vi "config.vi"() -> ()   [LabVIEW 2013]
uses:
  <vilib>/Utility/config.llb/NI_LVConfig.lvlib
panel:
  in  "选项卡控件":enum32{"操作步骤", "产品管理"}(tab)
  in  "第二段":T1
  in  "参数设定":string[][](table)
  in  "删除":bool
  in  "确定":bool
  in  "添加":bool
  in  "退出":bool
  in  "更新":bool
  in  "产品型号":string(combo)
  in  "操作步骤":T2
  in  "请输入添加的产品名称":string
  in  "请选择要删除的产品":string(combo)
  # "出厂检验台"
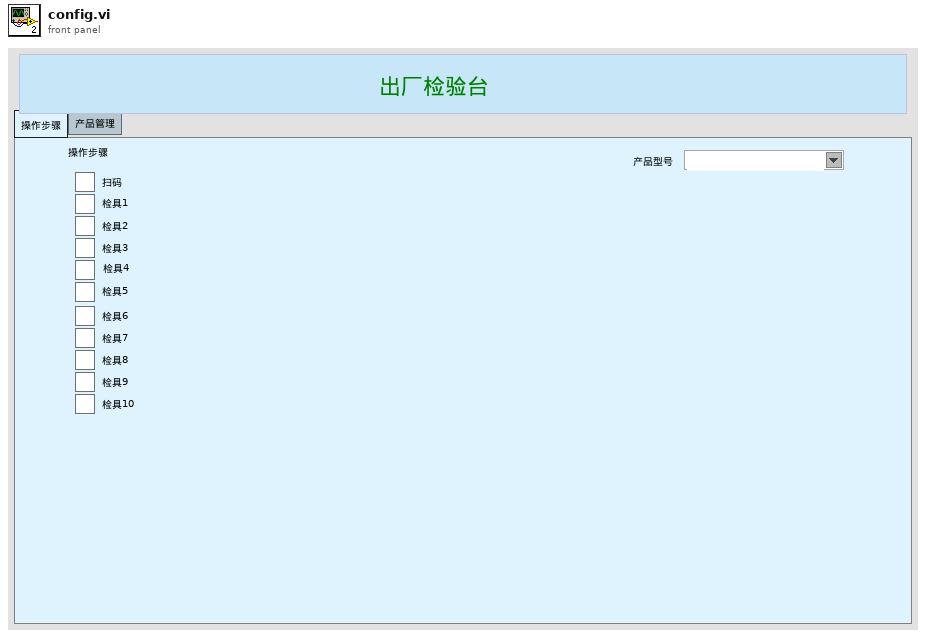
[diagram p1: front panel]
types:
  T1 = cluster{"检具6":bool, "检具7":bool, "检具8":bool, "检具9":bool, "检具10":bool}
  T2 = cluster{"扫码":bool, "检具1":bool, "检具2":bool, "检具3":bool, bool, "检具5":bool}
  T3 = typedef "NI_LVConfig.lvlib/Config Data RefNum.ctl" = refnum<k1>
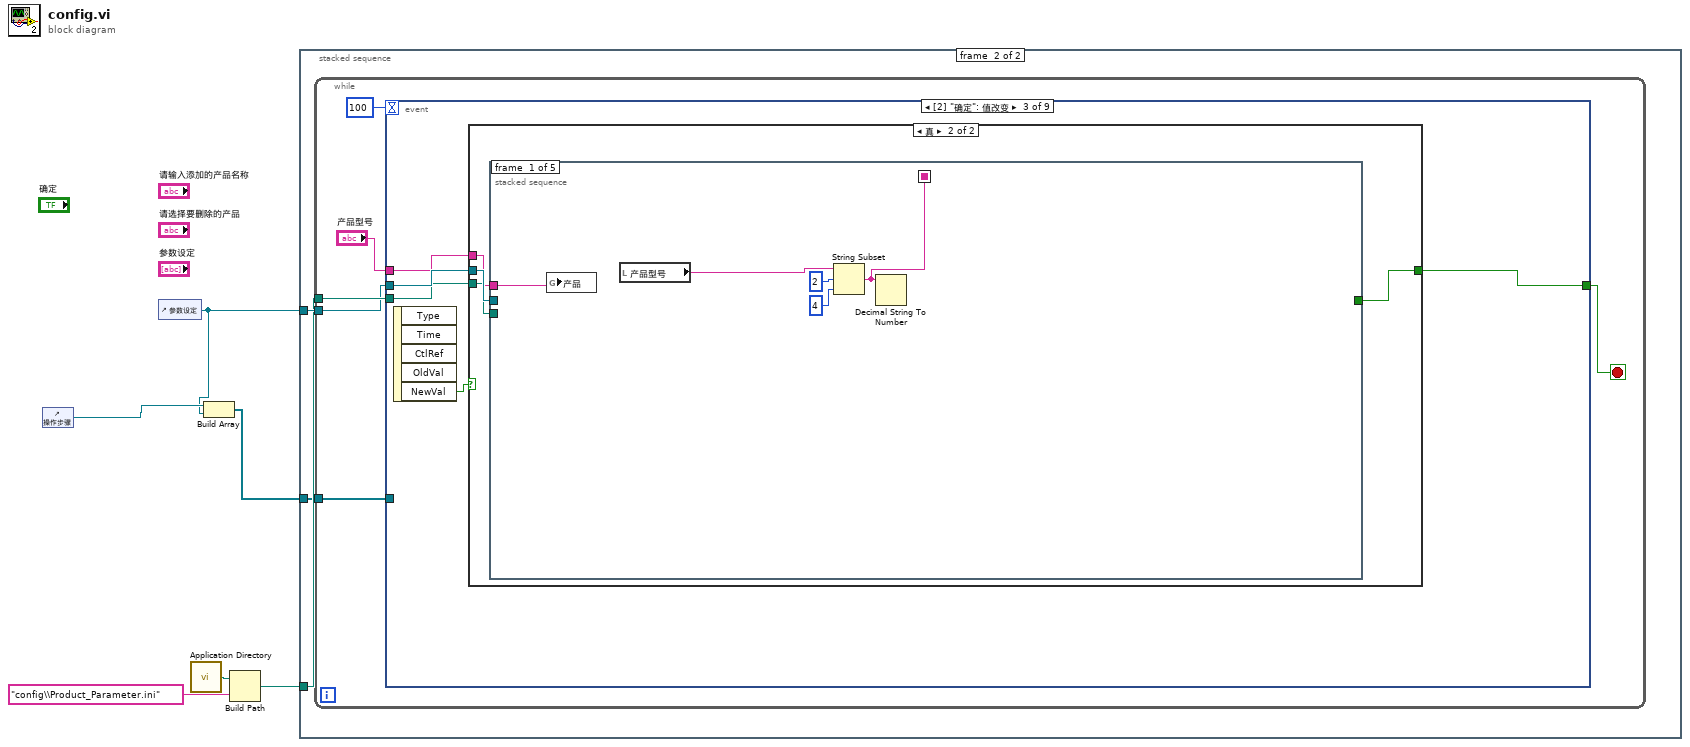
[diagram p0: block diagram]
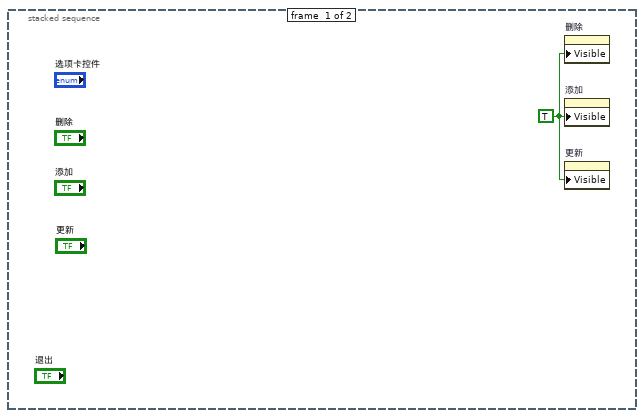
[diagram p2: hidden frame]
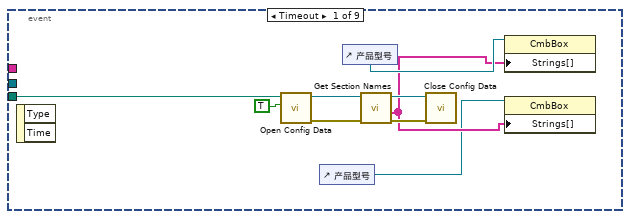
[diagram p3: hidden frame]
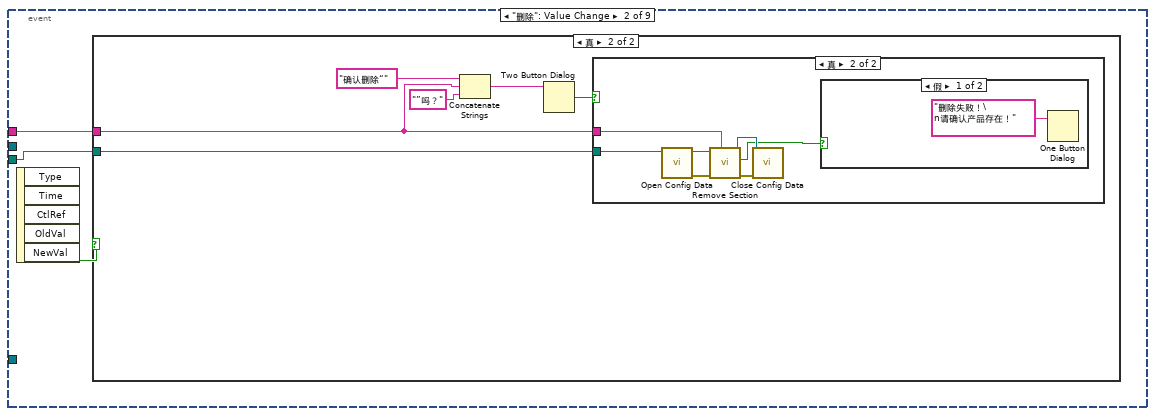
[diagram p4: hidden frame]
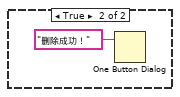
[diagram p7: hidden frame]
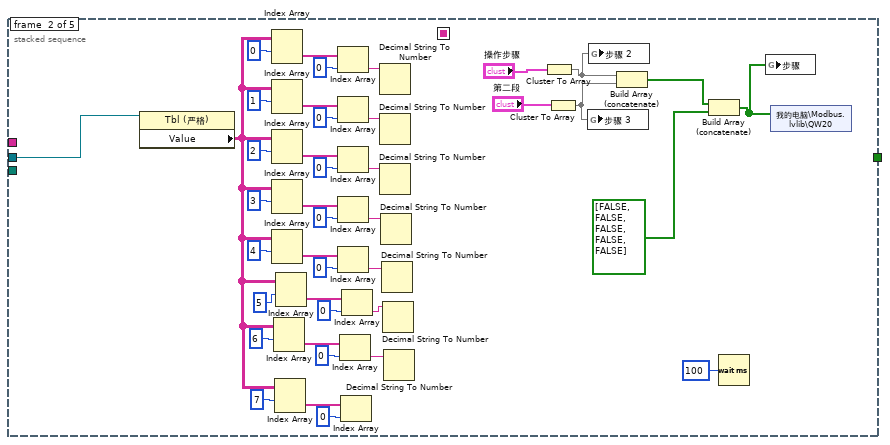
[diagram p9: hidden frame]
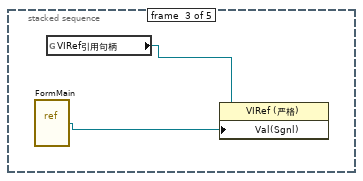
[diagram p10: hidden frame]
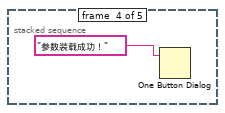
[diagram p11: hidden frame]
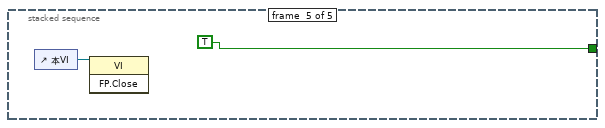
[diagram p12: hidden frame]
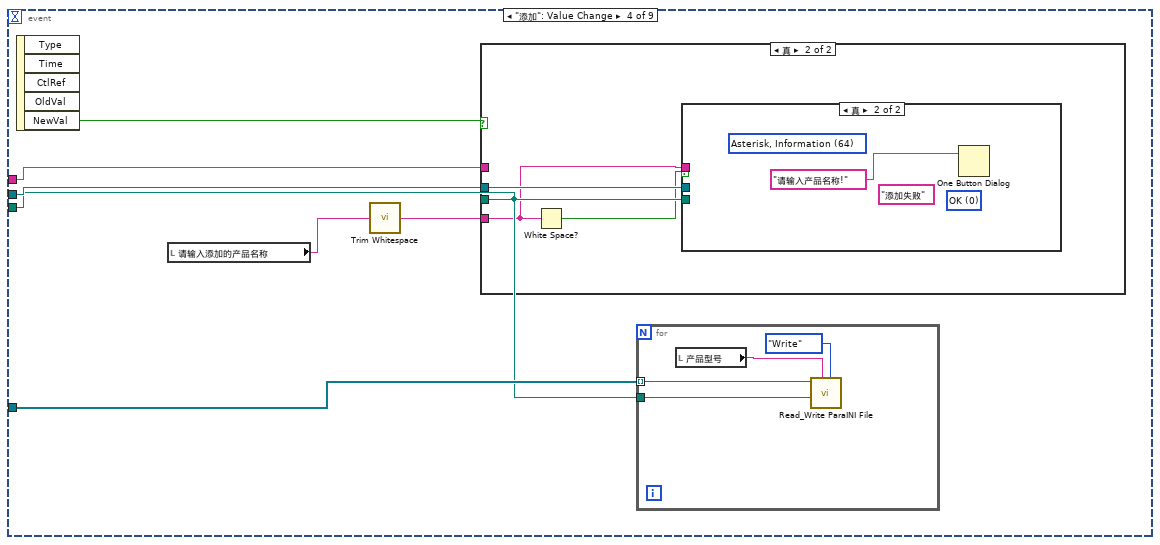
[diagram p13: hidden frame]
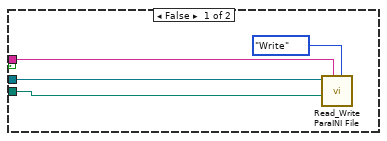
[diagram p15: hidden frame]
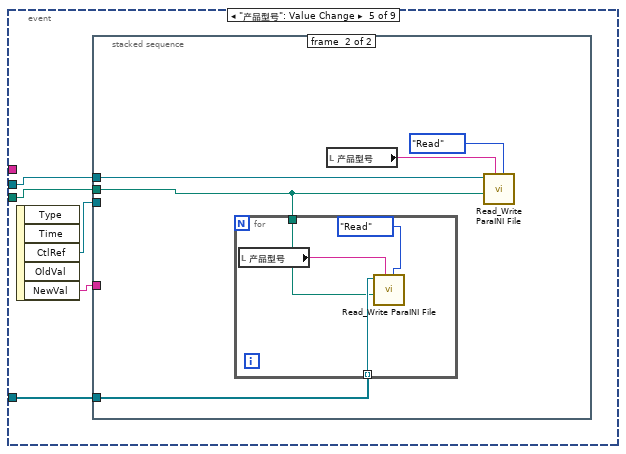
[diagram p16: hidden frame]
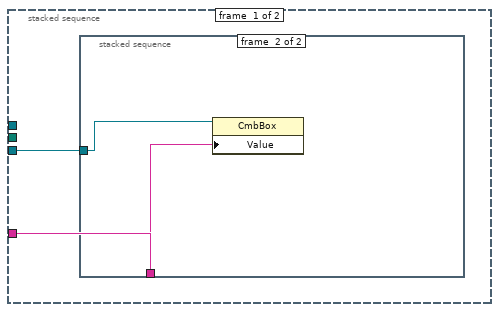
[diagram p17: hidden frame]
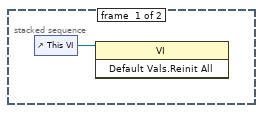
[diagram p18: hidden frame]
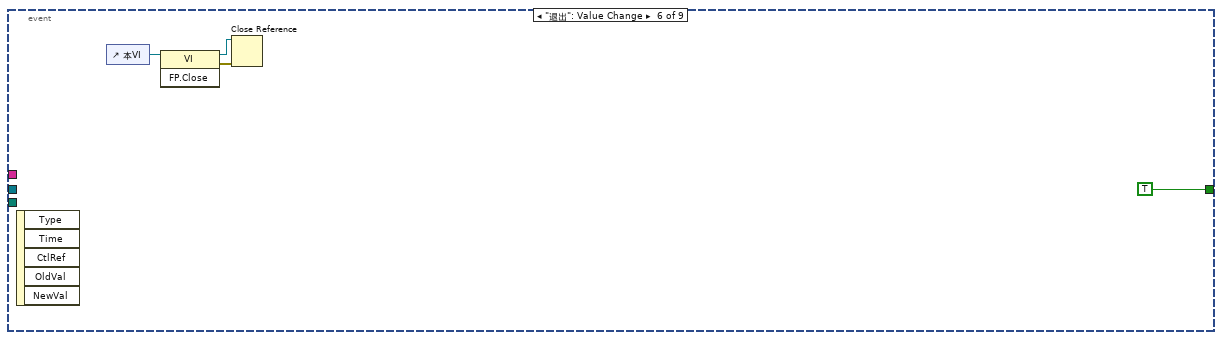
[diagram p19: hidden frame]
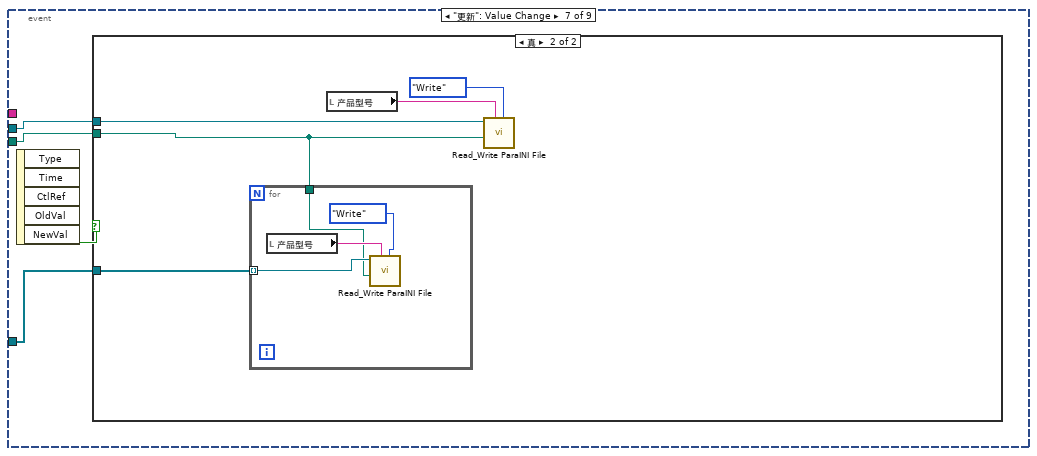
[diagram p20: hidden frame]
diagram:
  n1 = control-ref of="操作步骤"() -> (w3:refnum<vi>)
  n2 = control-ref of="参数设定"() -> (w1:refnum<vi>)
  n3 = call <vilib>:"Application Directory.vi"() -> ("Application Directory"=w6:path)
  n4 = Build Array(w3, w1) -> (w2:refnum<vi>[])
  n5 = Build Path(base path=w6, name or relative path="config\\Product_Parameter.ini" ("名称或相对路径")) -> (appended path=w4:path)
  n6 = stacked-sequence {
    tunnel: w1 -> [_ w10]
    tunnel: w4 -> [_ w9]
    tunnel: w2 -> [_ w8]
    frame #0 {
      w7 = TRUE ("可见")
      n7 = property on="删除" class="Bool (严格)"("Visible"=w7) -> ()  [unwired: 2 in, 2 out]
      n8 = property on="添加" class="Bool (严格)"("Visible"=w7) -> ()  [unwired: 2 in, 2 out]
      n9 = property on="更新" class="Bool (严格)"("Visible"=w7) -> ()  [unwired: 2 in, 2 out]
    }
    frame #1 {
      n10 = while {
        tunnel: w9 -> [w16]
        tunnel: w10 -> [w14]
        tunnel: w8 -> [w11]
        stop <- w15 stop-if-true
        n11 = event shown="[2] \"确定\": 值改变" {
          selector: _ -> [_ _ _ _ _ _ _ _ _]
          dyn-events: _ -> [_ _ _ _ _ _ _ _ _]
          timeout: 100 -> [_ _ _ _ _ _ _ _ _]
          tunnel: w16 -> [w20 w28 w45 w107 w127 _ w150 _ _]
          tunnel: [_ _ w47 _ _ TRUE _ _ TRUE] -> w15
          tunnel: w14 -> [_ _ w46 w110 w128 _ w149 _ _]
          tunnel: "产品型号" -> [_ w26 w44 w109 _ _ _ _ _]
          tunnel: w11 -> [_ _ _ w108 w124 _ w147 _ _]
          event Timeout {
            n12 = event-data() -> ()  [unwired: 1 in, 2 out]
            n13 = call <vilib>:"Open Config Data.vi"("create file if necessary (T)"=TRUE, "configuration file path"=w20) -> ("error out"=w22:errorcluster, "refnum"=w21:T3)  [unwired: 7 in, 1 out]
            n14 = control-ref of="产品型号"() -> (w17:refnum<vi>)
            n15 = control-ref of="产品型号"() -> (w19:refnum<vi>)
            n16 = call <vilib>:"Get Section Names.vi"("error in (no error)"=w22, "refnum"=w21) -> ("error out"=w24:errorcluster, "section names"=w18:string[], "refnum out"=w23:T3)  [unwired: 7 in]
            n17 = call <vilib>:"Close Config Data.vi"("error in (no error)"=w24, "refnum"=w23) -> ()  [unwired: 8 in, 2 out]
            n18 = property on="属性节点" class="CmbBox"(reference=w19, "Strings[]"=w18) -> ()  [unwired: 1 in, 2 out]
            n19 = property on="属性节点" class="CmbBox"(reference=w17, "Strings[]"=w18) -> ()  [unwired: 1 in, 2 out]
          }
          event "删除": Value Change {
            n20 = event-data() -> ("NewVal"=w27:bool)  [unwired: 1 in, 4 out]
            n21 = case shown="真" w27 {
              tunnel: w28 -> [_ w30]
              tunnel: w26 -> [_ w29]
              frame False {
              }
              frame True {
                n22 = Concatenate Strings("确认删除“", w29, "”吗？") -> (w32:string)
                n23 = Two Button Dialog(message=w32) -> (T button?=w31:bool)  [unwired: 2 in]
                n24 = case shown="真" w31 {
                  tunnel: w30 -> [_ w36]
                  tunnel: w29 -> [_ w35]
                  frame False {
                  }
                  frame True {
                    n25 = call <vilib>:"Open Config Data.vi"("configuration file path"=w36) -> ("error out"=w38:errorcluster, "refnum"=w41:T3)  [unwired: 8 in, 1 out]
                    n26 = call <vilib>:"Remove Section.vi"("section"=w35, "error in (no error)"=w38, "refnum"=w41) -> ("error out"=w40:errorcluster, "section exists?"=w37:bool, "refnum out"=w39:T3)  [unwired: 6 in]
                    n27 = call <vilib>:"Close Config Data.vi"("error in (no error)"=w40, "refnum"=w39) -> ()  [unwired: 8 in, 2 out]
                    n28 = case shown="假" w37 {
                      frame False {
                        n29 = One Button Dialog(message="删除失败！\n请确认产品存在！" ("消息")) -> ()  [unwired: 1 in, 1 out]
                      }
                      frame True {
                        n30 = One Button Dialog(message="删除成功！" ("消息")) -> ()  [unwired: 1 in, 1 out]
                      }
                    }
                  }
                }
              }
            }
          }
          event "确定": Value Change {
            n31 = event-data() -> ("NewVal"=w48:bool)  [unwired: 1 in, 4 out]
            n32 = case shown="真" w48 {
              tunnel: [_ w52] -> w47
              tunnel: w46 -> [_ w51]
              tunnel: w45 -> [_ w50]
              tunnel: w44 -> [_ w49]
              frame False {
              }
              frame True {
                n33 = stacked-sequence {
                  seq-local: [w57 _ _ _ _] -> [_ _ _ _ _]
                  tunnel: [_ _ _ _ TRUE] -> w52
                  tunnel: w51 -> [_ w64 _ _ _]
                  tunnel: w50 -> [_ _ _ _ _]
                  tunnel: w49 -> [w53 _ _ _ _]
                  frame #0 {
                    n34 = global write "全局 3.vi" "产品"(w53) -> ()
                    n35 = local read "产品型号"() -> (w56:string)
                    n36 = String Subset(string=w56, offset (0)=u16 2 ("偏移量(0)"), length (rest)=u16 4 ("长度（剩余）")) -> (substring=w57:string)
                    n37 = Decimal String To Number(string=w57) -> ()  [unwired: 2 in, 2 out]
                  }
                  frame #1 {
                    n38 = property class="Tbl (严格)"(reference=w64) -> ("Value"=w66:string[][])  [unwired: 1 in, 2 out]
                    n39 = Index Array(array=w66, index (row)=0 ("索引 (行)")) -> (element=w96:string[])  [unwired: 1 in]
                    n40 = Index Array(array=w66, index (row)=1 ("索引 (行)")) -> (element=w85:string[])  [unwired: 1 in]
                    n41 = Index Array(array=w66, index (row)=2 ("索引 (行)")) -> (element=w84:string[])  [unwired: 1 in]
                    n42 = Index Array(array=w66, index (row)=3 ("索引 (行)")) -> (element=w80:string[])  [unwired: 1 in]
                    n43 = Index Array(array=w66, index (row)=4 ("索引 (行)")) -> (element=w81:string[])  [unwired: 1 in]
                    n44 = Index Array(array=w66, index (row)=6 ("索引 (行)")) -> (element=w76:string[])  [unwired: 1 in]
                    n45 = Index Array(array=w66, index (row)=7 ("索引 (行)")) -> (element=w67:string[])  [unwired: 1 in]
                    n46 = Index Array(array=w66, index (row)=5 ("禁用的索引 (列)")) -> (element=w73:string[])  [unwired: 1 in]
                    n47 = Index Array(array=w96, index=0 ("索引")) -> (element=w97:string)
                    n48 = Index Array(array=w85, index=0 ("索引")) -> (element=w88:string)
                    n49 = Index Array(array=w84, index=0 ("索引")) -> (element=w87:string)
                    n50 = Index Array(array=w80, index=0 ("索引")) -> (element=w79:string)
                    n51 = Index Array(array=w81, index=0 ("索引")) -> (element=w78:string)
                    n52 = Index Array(array=w76, index=0 ("索引")) -> (element=w77:string)
                    n53 = Index Array(array=w67, index=0 ("索引")) -> ()  [unwired: 1 out]
                    n54 = Index Array(array=w73, index=0 ("索引")) -> (element=w71:string)
                    n55 = Decimal String To Number(string=w97) -> ()  [unwired: 2 in, 2 out]
                    n56 = Decimal String To Number(string=w88) -> ()  [unwired: 2 in, 2 out]
                    n57 = Decimal String To Number(string=w87) -> ()  [unwired: 2 in, 2 out]
                    n58 = Decimal String To Number(string=w79) -> ()  [unwired: 2 in, 2 out]
                    n59 = Decimal String To Number(string=w78) -> ()  [unwired: 2 in, 2 out]
                    n60 = Decimal String To Number(string=w71) -> ()  [unwired: 2 in, 2 out]
                    n61 = Decimal String To Number(string=w77) -> ()  [unwired: 2 in, 2 out]
                    n62 = Cluster To Array(cluster="操作步骤") -> (array=w59:bool[])
                    n63 = Cluster To Array(cluster="第二段") -> (array=w58:bool[])
                    n64 = global write "全局 3.vi" "步骤 3"(w58) -> ()
                    n65 = global write "全局 3.vi" "步骤 2"(w59) -> ()
                    n66 = Build Array (concatenate)(w59, w58) -> (w61:bool[])
                    n67 = Build Array (concatenate)(w61, bool[] [FALSE, FALSE, FALSE, FALSE, FALSE] ("数组")) -> (w60:bool[])
                    n68 = Wait (ms)(milliseconds to wait=u32 100) -> ()  [unwired: 1 out]
                    n69 = global write "全局 3.vi" "步骤"(w60) -> ()
                    n70 = shared-variable "我的电脑\\Modbus.lvlib\\QW20"(w60) -> ()  [unwired: 1 in, 1 out]
                  }
                  frame #2 {
                    n71 = vi-ref "FormMain.vi"() -> (w100:refnum<vi>)
                    n72 = global read "全局 3.vi" "VIRef引用句柄"() -> (w99:refnum<vi>)
                    n73 = property class="VIRef (严格)"(reference=w99, "Val(Sgnl)"=w100) -> ()  [unwired: 1 in, 2 out]
                  }
                  frame #3 {
                    n74 = One Button Dialog(message="参数装载成功！" ("消息")) -> ()  [unwired: 1 in, 1 out]
                  }
                  frame #4 {
                    n75 = control-ref of="本VI"() -> (w102:refnum<vi>)
                    n76 = invoke class="VI" method="FP.Close"(reference=w102) -> ()  [unwired: 2 in, 3 out]
                  }
                }
              }
            }
          }
          event "添加": Value Change {
            n77 = event-data() -> ("NewVal"=w106:bool)  [unwired: 1 in, 4 out]
            n78 = local read "请输入添加的产品名称"() -> (w105:string)
            n79 = call <vilib>:"Trim Whitespace.vi"("string"=w105) -> ("trimmed string"=w104:string)  [unwired: 1 in]
            n80 = case shown="真" w106 {
              tunnel: w110 -> [_ w118]
              tunnel: w107 -> [_ w117]
              tunnel: w109 -> [_ _]
              tunnel: w104 -> [_ w115]
              frame False {
              }
              frame True {
                n81 = White Space?(1:w115) -> (0:w116:bool)
                n82 = case shown="真" w116 {
                  tunnel: w118 -> [w122 _]
                  tunnel: w117 -> [w121 _]
                  tunnel: w115 -> [w120 _]
                  frame False {
                    n83 = call "Read_Write ParaINI File.vi"("Mode"=enum16{"Read", "Write"}."Write", "Section"=w120, "Filepath"=w121, "Ctl Refnum"=w122) -> ()  [unwired: 7 in, 1 out]
                  }
                  frame True {
                    (unwired) 64 items=["None"=0, "Hand, Error, Stop"=16, "Question"=32, "Exclamation, Warning"=48, "Asterisk, Information"=64] ("icon")
                    (unwired) 0 items=["OK", "OKCancel", "AbortRetryIgnore", "YesNoCancel", "YesNo", "RetryCancel"] ("buttons")
                    (unwired) "添加失败" ("caption")
                    n84 = One Button Dialog(message="请输入产品名称!" ("text")) -> ()  [unwired: 1 in, 1 out]
                  }
                }
              }
            }
            n85 = for {
              tunnel: w108 -> [w112] mode=indexing
              tunnel: w107 -> [w111]
              n86 = local read "产品型号"() -> (w113:string)
              n87 = call "Read_Write ParaINI File.vi"("Mode"=enum16{"Read", "Write"}."Write", "Section"=w113, "Filepath"=w111, "Ctl Refnum"=w112) -> ()  [unwired: 7 in, 1 out]
            }
          }
          event "产品型号": Value Change {
            n88 = event-data() -> ("CtlRef"=w126:refnum<vi>, "NewVal"=w125:string)  [unwired: 1 in, 3 out]
            n89 = stacked-sequence {
              tunnel: w128 -> [_ w138]
              tunnel: w127 -> [_ w134]
              tunnel: w126 -> [w130 _]
              tunnel: w125 -> [w129 _]
              tunnel: w124 -> [_ w135]
              frame #0 {
                n90 = stacked-sequence {
                  tunnel: w130 -> [_ w132]
                  tunnel: w129 -> [_ w133]
                  frame #0 {
                    n91 = control-ref of="This VI"() -> (w131:refnum<vi>)
                    n92 = invoke class="VI" method="Default Vals.Reinit All"(reference=w131) -> ()  [unwired: 2 in, 3 out]
                  }
                  frame #1 {
                    n93 = property class="CmbBox"(reference=w132, "Value"=w133) -> ()  [unwired: 1 in, 2 out]
                  }
                }
              }
              frame #1 {
                n94 = for {
                  tunnel: w135 -> [w141] mode=indexing
                  tunnel: w134 -> [w140]
                  n95 = local read "产品型号"() -> (w139:string)
                  n96 = call "Read_Write ParaINI File.vi"("Mode"=enum16{"Read", "Write"}."Read", "Section"=w139, "Filepath"=w140, "Ctl Refnum"=w141) -> ()  [unwired: 7 in, 1 out]
                }
                n97 = local read "产品型号"() -> (w136:string)
                n98 = call "Read_Write ParaINI File.vi"("Mode"=enum16{"Read", "Write"}."Read", "Section"=w136, "Filepath"=w134, "Ctl Refnum"=w138) -> ()  [unwired: 7 in, 1 out]
              }
            }
          }
          event "退出": Value Change {
            n99 = event-data() -> ()  [unwired: 1 in, 5 out]
            n100 = control-ref of="本VI"() -> (w145:refnum<vi>)
            n101 = invoke class="VI" method="FP.Close"(reference=w145) -> (reference out=w143:refnum<vi>, error out=w144:errorcluster)  [unwired: 2 in, 1 out]
            n102 = Close Reference(reference=w143, error in (no error)=w144) -> ()  [unwired: 1 out]
          }
          event "更新": Value Change {
            n103 = event-data() -> ("NewVal"=w148:bool)  [unwired: 1 in, 4 out]
            n104 = case shown="真" w148 {
              tunnel: w150 -> [_ w151]
              tunnel: w149 -> [_ w155]
              tunnel: w147 -> [_ w152]
              frame False {
              }
              frame True {
                n105 = for {
                  tunnel: w152 -> [w157] mode=indexing
                  tunnel: w151 -> [w156]
                  n106 = local read "产品型号"() -> (w158:string)
                  n107 = call "Read_Write ParaINI File.vi"("Mode"=enum16{"Read", "Write"}."Write", "Section"=w158, "Filepath"=w156, "Ctl Refnum"=w157) -> ()  [unwired: 7 in, 1 out]
                }
                n108 = local read "产品型号"() -> (w154:string)
                n109 = call "Read_Write ParaINI File.vi"("Mode"=enum16{"Read", "Write"}."Write", "Section"=w154, "Filepath"=w151, "Ctl Refnum"=w155) -> ()  [unwired: 7 in, 1 out]
              }
            }
          }
          event "请输入添加的产品名称": Value Change {
            n110 = event-data() -> ("OldVal"=w162:string)  [unwired: 1 in, 5 out]
            n111 = control-ref of="产品型号"() -> (w160:refnum<vi>)
            n112 = property on="属性节点" class="CmbBox"(reference=w160) -> ("Strings[]"=w161:string[])  [unwired: 1 in, 2 out]
            n113 = for {
              tunnel: w162 -> [w163]
              tunnel: w161 -> [w164] mode=indexing
              n114 = Equal?(x=w163, y=w164) -> (x = y?=w165:bool)
              n115 = case shown="真" w165 {
                tunnel: w163 -> [_ w166]
                frame False {
                }
                frame True {
                  n116 = stacked-sequence {
                    tunnel: w166 -> [w169 _]
                    frame #0 {
                      (unwired) 64 items=["None"=0, "Hand, Error, Stop"=16, "Question"=32, "Exclamation, Warning"=48, "Asterisk, Information"=64] ("icon")
                      n117 = Concatenate Strings("已经存在产品”" ("text"), w169, "“\n请勿重复添加！" ("字符串")) -> (w167:string)
                      n118 = One Button Dialog(message=w167) -> ()  [unwired: 1 in, 1 out]
                    }
                    frame #1 {
                      n119 = local write "请输入添加的产品名称"("" ("请输入添加的产品名称")) -> ()
                    }
                  }
                }
              }
            }
          }
          event Panel Close {
            n120 = event-data() -> ()  [unwired: 1 in, 3 out]
          }
        }
      }
    }
  }
